vi "CameraSetTimeout.vi"(8 "error in (no error)":errorcluster, 10 "Timeout":u32, 11 "AndorSDK3 in":refnum<class "Andor3.lvclass">) -> (0 "error out":errorcluster, 2 "Timeout set":u32, 3 "AndorSDK3 out":refnum<class "Andor3.lvclass">)   [LabVIEW 2010, in "Andor3.lvclass"]
uses:
  Andor3.lvclass
  Andor3.lvclass/Andor3.ctl
panel:
  # "Camera Configuration"
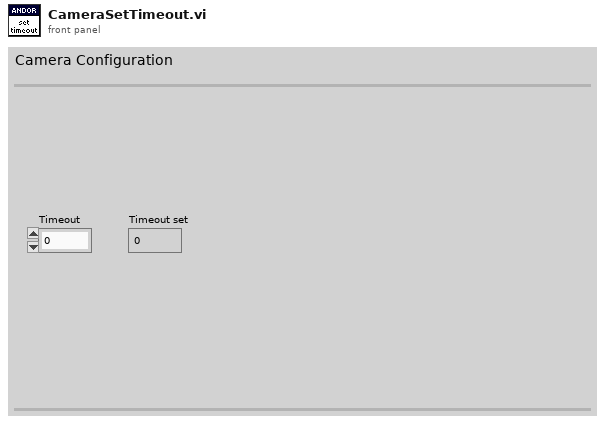
[diagram p1: front panel]
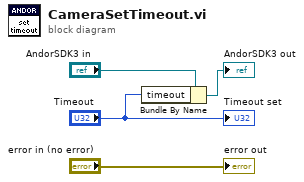
[diagram p0: block diagram]
diagram:
  n1 = Bundle By Name(cluster="AndorSDK3 in", "timeout"="Timeout") -> (→"AndorSDK3 out":refnum<class "Andor3.lvclass">)
  "error out" <- "error in (no error)"
  "Timeout set" <- "Timeout"
